vi "ClassLoader.vi"() -> (0 "ClassLoader":refnum<class "ClassLoader.lvclass">)   [LabVIEW 2020, in "ClassLoader_VIMs.lvlib"]
uses:
  ClassLoader_VIMs.lvlib
  ClassLoader/ClassLoader.lvclass
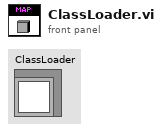
[diagram p1: front panel]
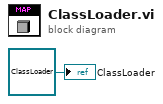
[diagram p0: block diagram]
diagram:
  "ClassLoader" <- refnum<class "ClassLoader.lvclass"> refnum ("ClassLoader.lvlib:ClassLoader.lvclass")
